vi "Micro-Epsilon ILD1420.vi"() -> (0 "DAQ Error":errorcluster)   [LabVIEW 2020]
uses:
  Globals/Meas_global.vi
  <vilib>/Instr/_visa.llb/VISA Find Search Mode.ctl
  Sub_vis/Upload Data.ctl
panel:
  out "Data Rate Hz":dbl
  out "Waveform Graph":cluster{"y":dbl, dbl, "d (mm)":dbl[]}(graph)
  in  "Reconfigure settings":bool
  out "Data rate (kHz)":string(combo)="0.25"
  out "Measuring range (mm)":u8(ring)=4 items=["10", "25", "50", "100", "200"]
  in  "Auto laser off":bool=TRUE
  # "(set true if changing data rate)"
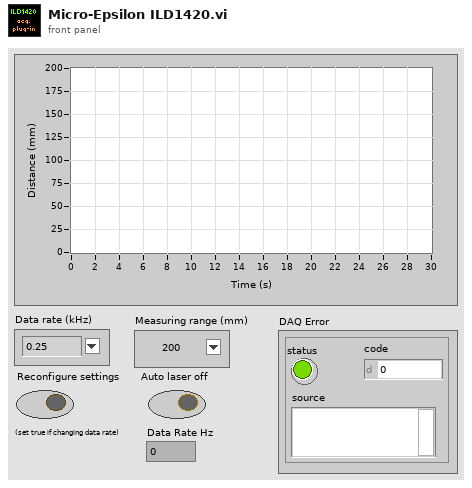
[diagram p1: front panel]
types:
  T1 = typedef "Setup.ctl" = enum16{"Run Program", "Show Setup", "Save Current Setup", "Setup Front Panel"}
  T2 = typedef "Upload Data.ctl" = enum16{"Voltage Array", "Time Trace Cluster"}
  T3 = typedef "VISA Find Search Mode.ctl" = u32
  T4 = typedef "Rendezvous RefNum" = refnum<k1>
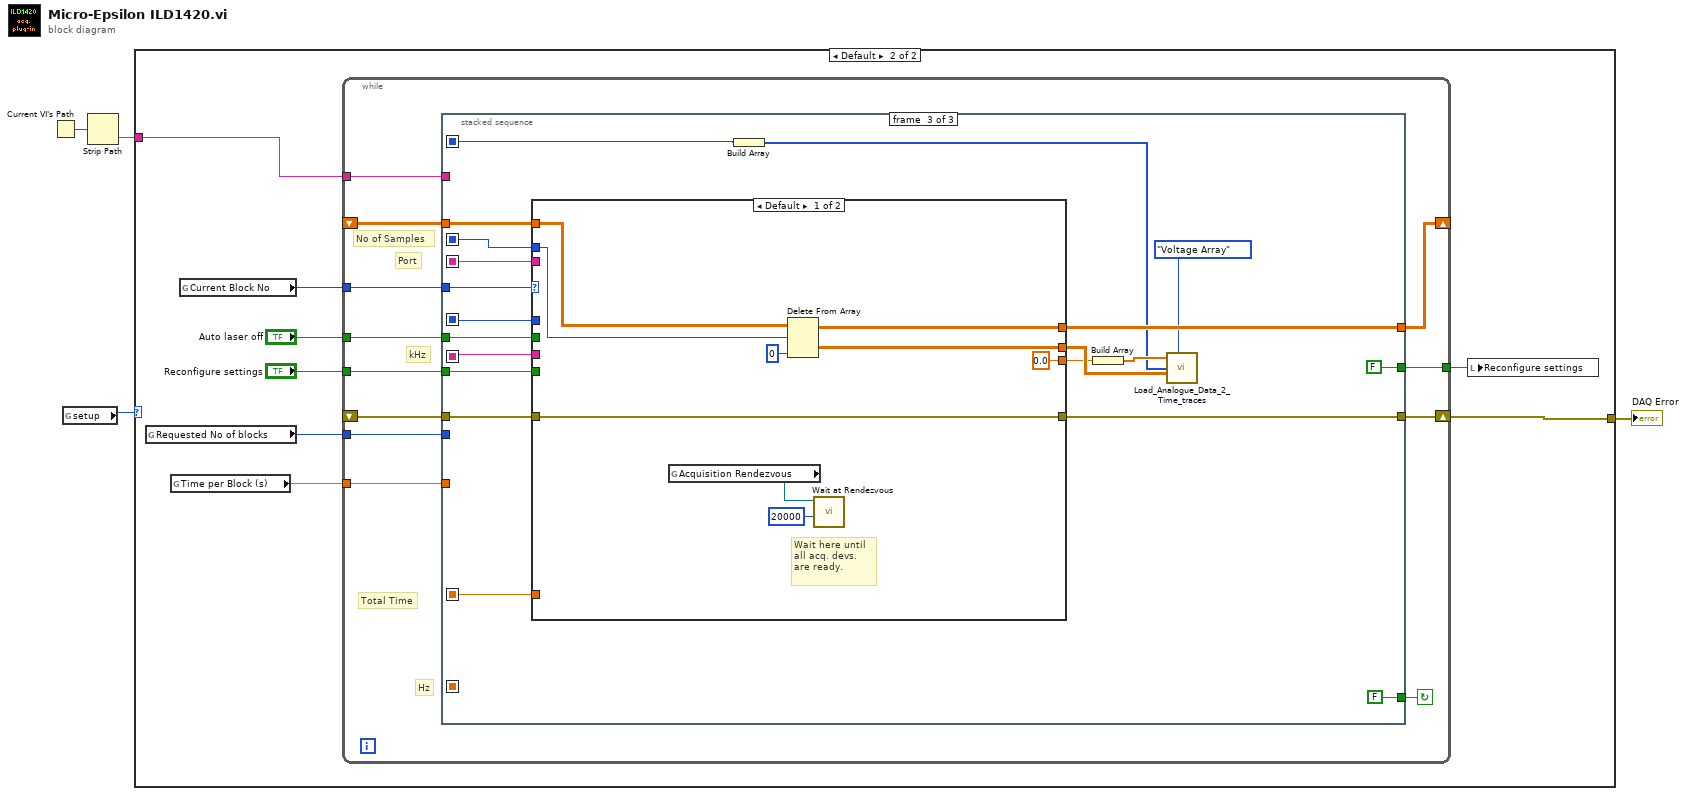
[diagram p0: block diagram]
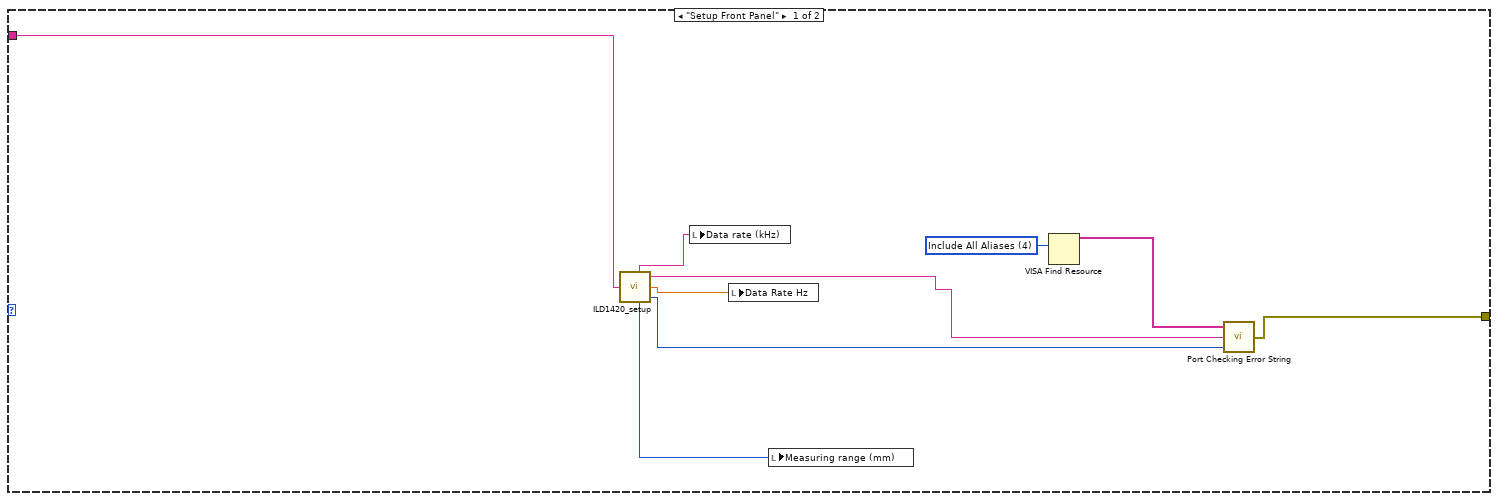
[diagram p2: hidden frame]
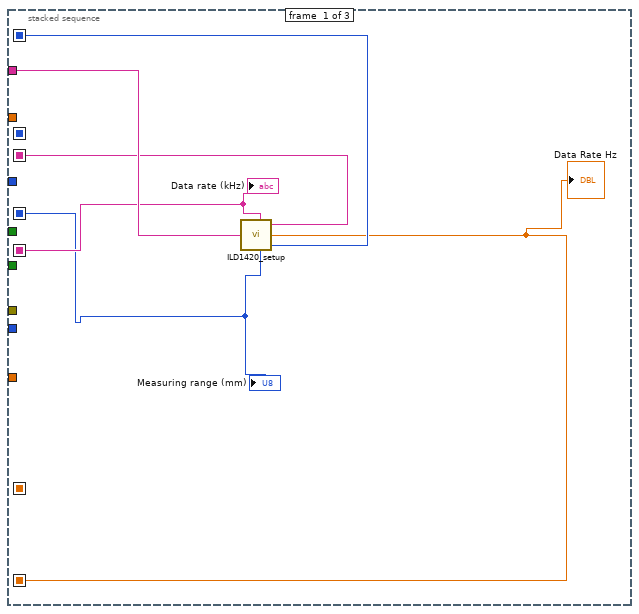
[diagram p3: hidden frame]
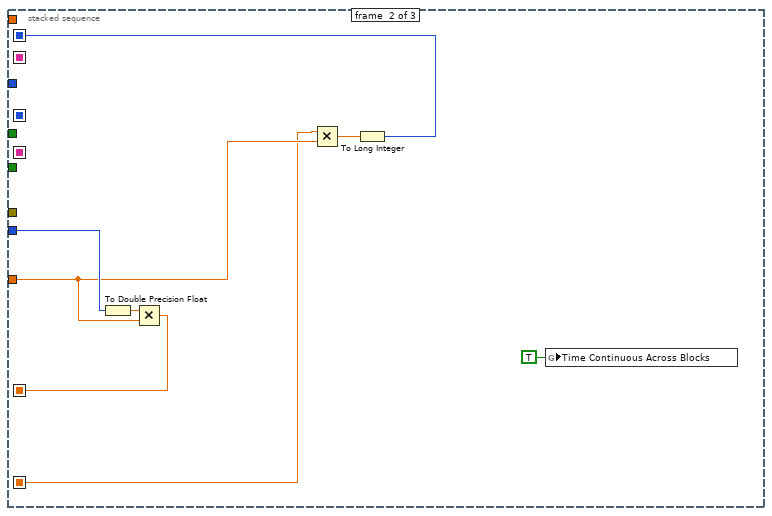
[diagram p4: hidden frame]
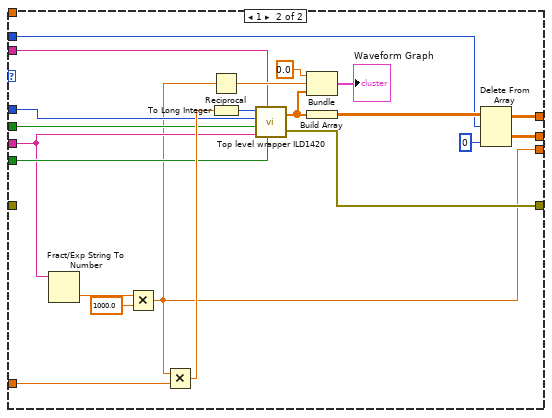
[diagram p5: hidden frame]
diagram:
  n1 = Current VI's Path() -> (path=w2:path)
  n2 = global read "Meas_global.vi" "setup"() -> (w3:T1)
  n3 = Strip Path(path=w2) -> (name=w1:string)  [unwired: 1 out]
  n4 = case shown="Default" w3 {
    tunnel: [w11 w19] -> w4
    tunnel: w1 -> [w10 w14]
    frame "Setup Front Panel" {
      w13 = T3 4 items=["Canonical Names Only"=0, "Aliases Only"=1, "Include Matching Aliases"=2, "Include All Aliases"=4] ("Search Mode")
      n5 = call "ILD1420_setup.vi"("Device Name"=w10) -> ("Index"=w8:i32, "Measuring range (mm)"=w5:u8, "Data Rate Hz"=w7:dbl, "Port"=w9:string, "Data rate (kHz)"=w6:string)
      n6 = local write "Data rate (kHz)"(w6) -> ()
      n7 = local write "Data Rate Hz"(w7) -> ()
      n8 = local write "Measuring range (mm)"(w5) -> ()
      n9 = VISA Find Resource(10:w13) -> (3:w12:string[])  [unwired: 2 in, 2 out]
      n10 = call "Port Checking Error String.vi"("Ch Index"=w8, "Port"=w9, "Available Ports"=w12) -> ("error out"=w11:errorcluster)  [unwired: 1 in]
    }
    frame Default {
      n11 = global read "Meas_global.vi" "Requested No of blocks"() -> (w20:i32)
      n12 = global read "Meas_global.vi" "Time per Block (s)"() -> (w15:dbl)
      n13 = global read "Meas_global.vi" "Current Block No"() -> (w21:i32)
      n14 = while {
        tunnel: w21 -> [w33]
        tunnel: w20 -> [w32]
        tunnel: "Auto laser off" -> [w30]
        shift-right: [w26] -> _
        shift-left: _ -> [w24]
        tunnel: "Reconfigure settings" -> [w29]
        tunnel: [w28] -> w16
        shift-right: [w31] -> w19
        shift-left: _ -> [w25]
        tunnel: w15 -> [w23]
        tunnel: w14 -> [w22]
        stop <- w27 continue-if-true
        # "Hz"
        # "kHz"
        # "Port"
        # "Total Time"
        # "No of Samples"
        n15 = stacked-sequence {
          seq-local: [_ w46 _] -> [_ _ w67]
          seq-local: [_ w41 _] -> [_ _ w54]
          seq-local: [w38 _ _] -> [_ _ w53]
          seq-local: [w36 _ _] -> [_ _ w51]
          seq-local: [w35 _ _] -> [_ _ w50]
          seq-local: [w34 _ _] -> [_ _ w49]
          seq-local: [w37 _ _] -> [_ w40 _]
          tunnel: w33 -> [_ _ w62]
          tunnel: w32 -> [_ w47 _]
          tunnel: [_ _ w66] -> w31
          tunnel: w30 -> [_ _ w65]
          tunnel: w29 -> [_ _ w64]
          tunnel: [_ _ FALSE ("Reconfigure settings")] -> w28
          tunnel: [_ _ FALSE ("Reconfigure settings")] -> w27
          tunnel: [_ _ w60] -> w26
          tunnel: w25 -> [_ _ w59]
          tunnel: w24 -> [_ _ w58]
          tunnel: w23 -> [_ w42 _]
          tunnel: w22 -> [w39 _ _]
          frame #0 {
            n16 = call "ILD1420_setup.vi"("Device Name"=w39) -> ("Index"=w38:i32, "Measuring range (mm)"=w34:u8, "Data Rate Hz"=w37:dbl, "Port"=w36:string, "Data rate (kHz)"=w35:string)
            "Data Rate Hz" <- w37
            "Data rate (kHz)" <- w35
            "Measuring range (mm)" <- w34
          }
          frame #1 {
            n17 = To Double Precision Float(number=w47) -> (double precision float=w44:dbl)
            n18 = Multiply(x=w44, y=w42) -> (x*y=w46:dbl)
            n19 = Multiply(x=w40, y=w42) -> (x*y=w43:dbl)
            n20 = To Long Integer(number=w43) -> (32bit integer=w41:i32)
            n21 = global write "Meas_global.vi" "Time Continuous Across Blocks"(TRUE ("Time Continuous across Blocks")) -> ()
          }
          frame #2 {
            n22 = case shown="Default" w62 {
              tunnel: w67 -> [_ w97]
              tunnel: [w76 w95] -> w66
              tunnel: w49 -> [_ w93]
              tunnel: w65 -> [_ w92]
              tunnel: w64 -> [_ w91]
              tunnel: w50 -> [_ w90]
              tunnel: [w72 w81] -> w57
              tunnel: w54 -> [w73 w80]
              tunnel: [w71 w79] -> w60
              tunnel: w59 -> [w76 _]
              tunnel: w58 -> [w74 _]
              tunnel: [0.0 w78] -> w56
              tunnel: w51 -> [_ w77]
              frame Default {
                # "Wait here until all acq. devs. are ready."
                n23 = global read "Meas_global.vi" "Acquisition Rendezvous"() -> (w69:T4)
                n24 = Delete From Array(array=w74, length=w73, index (col)=0 ("disabled index (col)")) -> (deleted portion=w72:dbl[][], array with subset deleted=w71:dbl[][])  [unwired: 1 in]
                n25 = call <vilib>:"Wait at Rendezvous.vi"("ms timeout (-1)"=20000, "rendezvous"=w69) -> ()  [unwired: 3 in, 3 out]
              }
              frame 1 {
                n26 = Fract/Exp String To Number(string=w90) -> (number=w89:dbl)  [unwired: 3 in, 1 out]
                n27 = Multiply(x=w89, y=1000.0) -> (x*y=w78:dbl)
                n28 = Multiply(x=w78, y=w97) -> (x*y=w96:dbl)
                n29 = Reciprocal(x=w78) -> (1/x=w85:dbl)
                n30 = To Long Integer(number=w96) -> (32bit integer=w94:i32)
                n31 = call "Top level wrapper ILD1420.vi"("Reconfigure settings"=w91, "ILD1420 COM port"=w77, "Data rate (kHz)"=w90, "Auto laser off"=w92, "Measuring range (mm)"=w93, "N samples"=w94) -> ("Error out"=w95:errorcluster, "d (mm)"=w87:dbl[])
                n32 = Bundle("y"=0.0, w85, "d (mm)"=w87) -> (→"Waveform Graph":cluster{"y":dbl, dbl, "d (mm)":dbl[]})  [unwired: 1 in]
                n33 = Build Array(w87) -> (w82:dbl[][])
                n34 = Delete From Array(array=w82, length=w80, index (col)=0 ("disabled index (col)")) -> (deleted portion=w81:dbl[][], array with subset deleted=w79:dbl[][])  [unwired: 1 in]
              }
            }
            n35 = Build Array(w53) -> (w52:i32[])
            n36 = Build Array(w56) -> (w55:dbl[])
            n37 = call "Load_Analogue_Data_2_Time_traces.vi"("Sampling Rate (Hz)"=w55, "Mode"=Upload_Data."Voltage Array", "Index"=w52, "Voltage Array"=w57) -> ()  [unwired: 3 in]
          }
        }
      }
      n38 = local write "Reconfigure settings"(w16) -> ()
    }
  }
  "DAQ Error" <- w4
